vi "updateDefaultSettings.vi"(1 "object":refnum<class>) -> ()   [LabVIEW 2017]
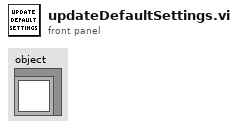
[diagram p1: front panel]
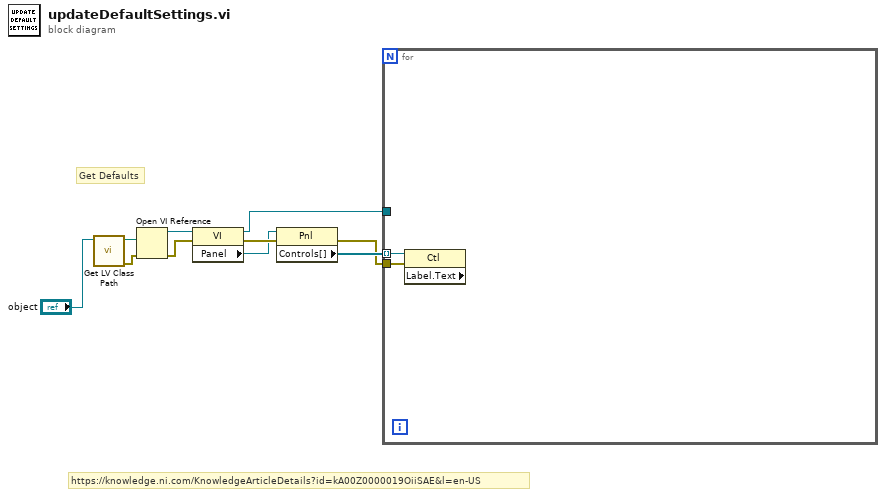
[diagram p0: block diagram]
diagram:
  # "Get Defaults"
  # "https://knowledge.ni.com/KnowledgeArticleDetails?id=kA00Z0000019OiiSAE&l=en-US"
  n1 = call <vilib>:"Get LV Class Path.vi"("object"="object") -> ("error out"=w7:errorcluster, "class path"=w10:path)  [unwired: 9 in]
  n2 = Open VI Reference(vi path=w10, error in (no error)=w7) -> (vi reference=w9:refnum<vi>, error out=w8:errorcluster)  [unwired: 4 in]
  n3 = property class="VI"(reference=w9, error in=w8) -> (reference out=w1:refnum<vi>, error out=w6:errorcluster, "Panel"=w5:refnum<vi>)
  n4 = property class="Pnl"(reference=w5, error in=w6) -> (error out=w2:errorcluster, "Controls[]"=w3:refnum<vi>[])  [unwired: 1 out]
  n5 = for {
    tunnel: w3 -> [w12] mode=indexing
    tunnel: w2 -> [w11]
    tunnel: w1 -> [_]
    n6 = property class="Ctl" props=["Label", "Text"](reference=w12, error in=w11) -> ()  [unwired: 3 out]
  }
